vi "VI Tree.vi"   [LabVIEW 2012, in "Phidget Digital Output.lvlib"]
doc: "${DigitalOutput:VITreeHeader}"
uses:
  <instrlib>/Phidgets/Phidget Digital Output/Phidget Digital Output.lvlib
  <instrlib>/Phidgets/Phidget Digital Output/Public/DigitalOutputStart.vi
  <instrlib>/Phidgets/Phidget Digital Output/Public/DigitalOutputOpen.vi
  <instrlib>/Phidgets/Phidget Digital Output/Public/DigitalOutputClose.vi
panel:
  # "(c) 2015 Phidgets Inc..  ALL RIGHTS RESERVED."
  # "SEE DIAGRAM\nFOR VI TREE."
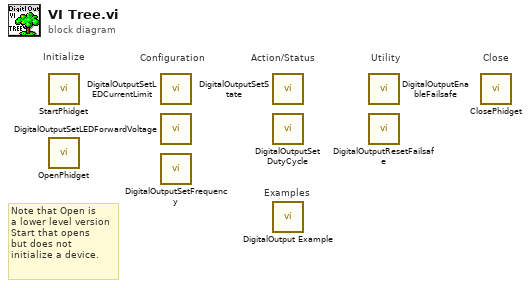
[diagram p0: block diagram]
diagram:
  # "Utility"
  # "Note that Open is\na lower level version\nStart that opens\nbut does not \ninitialize a device."
  # "Examples"
  # "Configuration"
  # "Action/Status"
  # "Close"
  # "Initialize"
  n1 = call-poly <instrlib>:"StartPhidget.vi"() -> ()  [unwired: 12 in, 4 out]
  n2 = call-poly <instrlib>:"OpenPhidget.vi"() -> ()  [unwired: 8 in, 4 out]
  n3 = call <instrlib>:"DigitalOutputSetLEDCurrentLimit.vi"() -> ()  [unwired: 9 in, 2 out]
  n4 = call <instrlib>:"DigitalOutputSetLEDForwardVoltage.vi"() -> ()  [unwired: 9 in, 2 out]
  n5 = call <instrlib>:"DigitalOutputSetFrequency.vi"() -> ()  [unwired: 9 in, 2 out]
  n6 = call <instrlib>:"DigitalOutputSetState.vi"() -> ()  [unwired: 9 in, 2 out]
  n7 = call <instrlib>:"DigitalOutputSetDutyCycle.vi"() -> ()  [unwired: 9 in, 2 out]
  n8 = call <instrlib>:"DigitalOutput Example.vi"() -> ()  [unwired: 12 in]
  n9 = call <instrlib>:"DigitalOutputEnableFailsafe.vi"() -> ()  [unwired: 9 in, 2 out]
  n10 = call <instrlib>:"DigitalOutputResetFailsafe.vi"() -> ()  [unwired: 9 in, 2 out]
  n11 = call-poly <instrlib>:"ClosePhidget.vi"() -> ()  [unwired: 11 in, 1 out]
